vi "RemoteControl.TestLauncher.Client4.vi"() -> ()   [LabVIEW 2016, in "RemoteControl.v2.lvclass"]
uses:
  RemoteControl.v2.lvclass
  <vilib>/JKI/JKI SMO/SMO/Typedefs/SMOState --Enum.ctl
  Typedefs/Message--Cluster.ctl
  C:/Program Files (x86)/National Instruments/LabVIEW 2016/vi.lib/JKI/JKI SMO/SMO/SMO.lvclass
  RemoteControl.STM/RemoteControl.STM.lvclass
  C:/user/patrick/hg/levylab_inst/lvsrc/SMOs/RemoteControl/RemoteControl.v2.lvclass
  Typedefs/PrivateEvents--RemoteControl.SendMessageToProcess.ctl
  <vilib>/JKI/JKI SMO/SMO/SMO.lvclass
panel:
  out "x-y":u32
  out "receive time":u32
  out "send time":u32
  in  "Send":bool
  out "received":i32
  out "sent":i32
  out "Message Sent":T1
  out "Message Received":T1
  in  "T = STM":bool
  in  "Message to Send":T1
  in  "Port":u32=6341
  in  "Address":string
  out "SMO State":T2
  out "error out":errorcluster
  in  "Stop":bool
  # "SM SMO Test Launcher: Client 4"
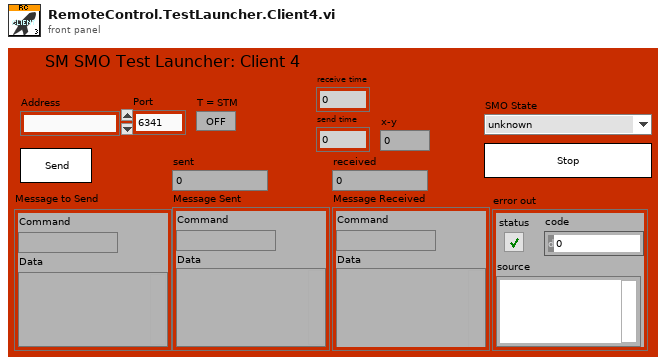
[diagram p1: front panel]
types:
  T1 = typedef "RemoteControl.v2.lvclass/Message--Cluster.ctl" = cluster{"Command":string, "Data":variant}
  T2 = typedef "SMO.lvclass/SMOState --Enum.ctl" = enum16{"unknown", "Created", "Started", "Stopped"}
  T3 = typedef "SMO.lvclass/Public Events.ctl" = cluster{"Error":refnum<user-event>, "State":refnum<user-event>, "Reserve State":refnum<user-event>}
  T4 = typedef "RemoteControl.v2.lvclass/PublicEvents--Cluster.ctl" = cluster{"SendMessageFromProcess":refnum<user-event>}
  T5 = typedef "RemoteControl.v2.lvclass/PrivateEvents--RemoteControl.SendMessageToProcess.ctl" = cluster{"Message":T1, "Message ID":u32}
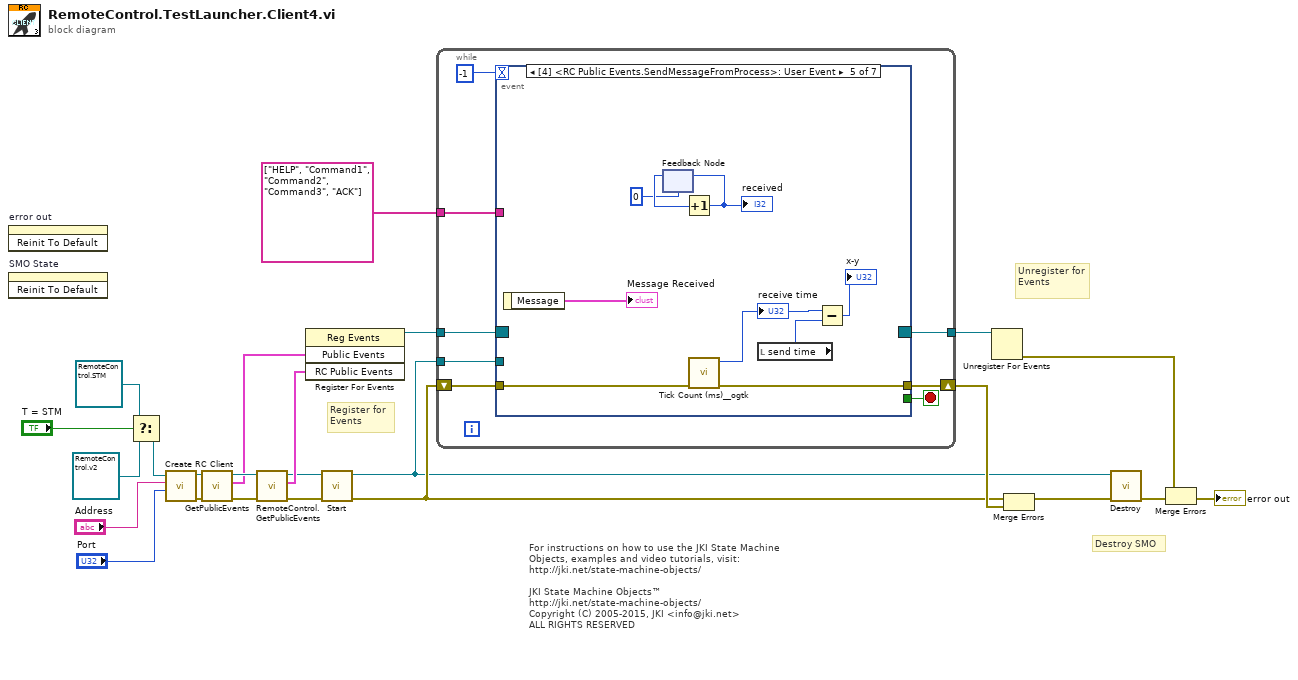
[diagram p0: block diagram]
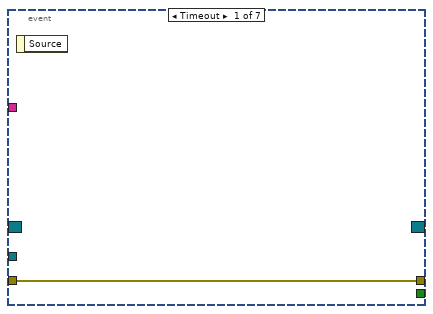
[diagram p2: hidden frame]
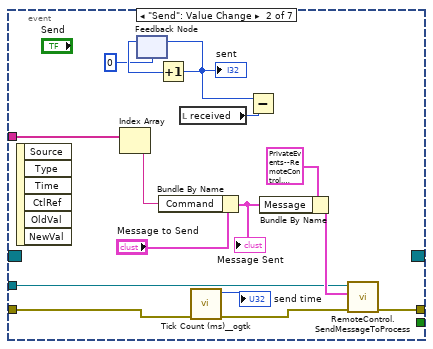
[diagram p3: hidden frame]
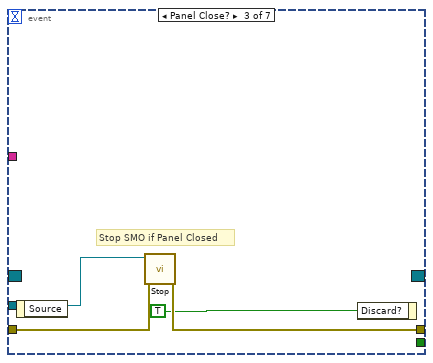
[diagram p4: hidden frame]
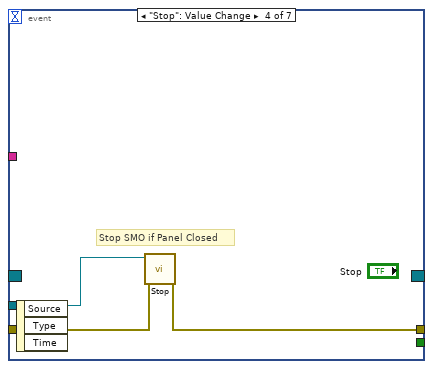
[diagram p5: hidden frame]
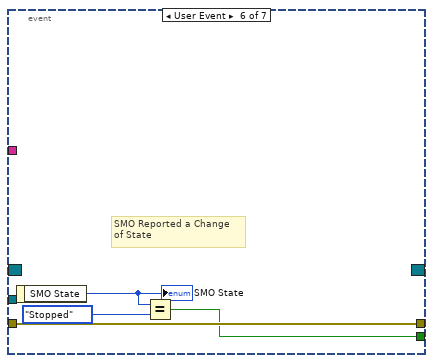
[diagram p6: hidden frame]
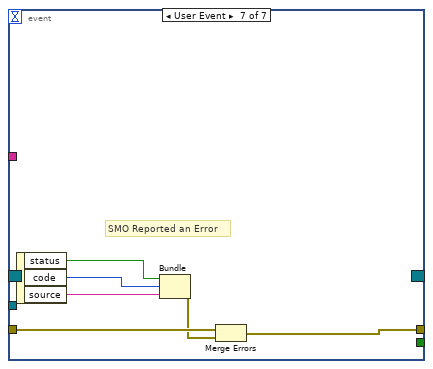
[diagram p7: hidden frame]
diagram:
  # "For instructions on how to use the JKI State Machine Objects, examples and video tutorials, visit:\nhttp://jki.net/state-machine-objects/\n\nJKI State Machine Objects™\nhttp://jki.net/state-machine-objects/\nCopyright (C) 2005-2015, JKI <info@jki.net>\nALL RIGHTS RESERVED"
  # "Destroy SMO"
  # "Unregister for Events"
  # "Register for Events"
  n1 = invoke on="error out" class="Clust (strict)" method="Reinit To Default"() -> ()  [unwired: 3 in, 3 out]
  n2 = invoke on="SMO State" class="Enum (strict)" method="Reinit To Default"() -> ()  [unwired: 3 in, 3 out]
  n3 = Select(t=refnum<class "RemoteControl.STM.lvclass"> refnum ("RemoteControl.STM.lvclass"), s="T = STM", f=refnum<class "RemoteControl.v2.lvclass"> refnum ("SMO.Template.lvclass")) -> (s? t:f=w13:refnum<class "RemoteControl.v2.lvclass">)
  n4 = call-dynamic "Create RC Client.vi"("Port"="Port", "Address"="Address", "RemoteControl in"=w13) -> ("error out"=w12:errorcluster, "RemoteControl out"=w11:refnum<class "RemoteControl.v2.lvclass">)  [unwired: 7 in]
  n5 = call <vilib>:"GetPublicEvents.vi"("error in (no error)"=w12, "SMO"=w11) -> ("error out"=w9:errorcluster, "Public Events"=w8:T3, "SMO out"=w10:refnum<class "RemoteControl.v2.lvclass">)  [unwired: 7 in]
  n6 = call "RemoteControl.GetPublicEvents.vi"("error in (no error)"=w9, "RemoteControl"=w10) -> ("error out"=w4:errorcluster, "RC Public Events"=w7:T4, "RemoteControl out"=w5:refnum<class "RemoteControl.v2.lvclass">)  [unwired: 7 in]
  n7 = register-events(w8, w7) -> (reference out=w6:refnum<event-registration>)  [unwired: 2 in, 1 out]
  n8 = call <vilib>:"Start.vi"("error in (no error)"=w4, "SMO"=w5) -> ("error out"=w3:errorcluster, "SMO out"=w2:refnum<class "RemoteControl.v2.lvclass">)  [unwired: 8 in]
  n9 = while {
    shift-right: [w31] -> w23
    shift-left: w3 -> [w30]
    tunnel: w6 -> [w29]
    tunnel: [w28] -> w24
    tunnel: w2 -> [w27]
    tunnel: string[] ["HELP", "Command1", "Command2", "Command3", "ACK"] ("Commands") -> [w26]
    stop <- w32 stop-if-true
    n10 = event shown="[4] <RC Public Events.SendMessageFromProcess>: User Event" {
      selector: w29 -> [_ _ _ _ _ _ _]
      dyn-events: [_ _ _ _ _ _ _] -> w28
      timeout: -1 -> [_ _ _ _ _ _ _]
      tunnel: [_ _ _ _ _ w65 _] -> w32
      tunnel: w27 -> [_ w38 w52 w55 _ _ _]
      tunnel: [w33 w39 w51 w54 w59 w68 w72] -> w31
      tunnel: w30 -> [w33 w36 w50 w53 w60 w68 w70]
      tunnel: w26 -> [_ w40 _ _ _ _ _]
      event Timeout {
        n11 = event-data() -> ()  [unwired: 1 in, 1 out]
      }
      event "Send": Value Change {
        n12 = event-data() -> ()  [unwired: 1 in, 6 out]
        n13 = Index Array(array=w40) -> (element=w37:string)  [unwired: 1 in]
        n14 = feedback #1(0) -> (w44:i32)
        n15 = Increment(x=w44) -> (x+1=w41:i32)
        "sent" <- w41
        n16 = feedback-in #1(w41) -> ()
        n17 = Bundle By Name(cluster="Message to Send", "Command"=w37) -> (w46:T1)
        "Message Sent" <- w46
        n18 = local read "received"() -> (w42:i32)
        n19 = call <userlib>:"Tick Count (ms)__ogtk.vi"("error in (no error)"=w36) -> ("error out"=w35:errorcluster, "millisecond timer value"=→"send time":u32)  [unwired: 9 in]
        n20 = Subtract(x=w41, y=w42) -> ()  [unwired: 1 out]
        n21 = Bundle By Name(cluster=T5 {"Message"={"Command"="", "Data"=variant(bool FALSE)}, "Message ID"=0} ("SendMessgaeToProcess"), "Message"=w46) -> (w47:T5)
        n22 = call "RemoteControl.SendMessageToProcess.vi"("error in (no error)"=w35, "SendMessgaeToProcess"=w47, "RemoteControl"=w38) -> ("error out"=w39:errorcluster)  [unwired: 7 in, 1 out]
      }
      event Panel Close? {
        # "Stop SMO if Panel Closed"
        n23 = event-data() -> ()  [unwired: 1 in, 1 out]
        n24 = call <vilib>:"Stop.vi"("error in (no error)"=w50, "SMO"=w52) -> ("error out"=w51:errorcluster)  [unwired: 8 in, 1 out]
        n25 = event-data("Discard?"=TRUE ("OK")) -> ()  [unwired: 1 in, 1 out]
      }
      event "Stop": Value Change {
        # "Stop SMO if Panel Closed"
        n26 = event-data() -> ()  [unwired: 1 in, 3 out]
        n27 = call <vilib>:"Stop.vi"("error in (no error)"=w53, "SMO"=w55) -> ("error out"=w54:errorcluster)  [unwired: 8 in, 1 out]
      }
      event User Event {
        n28 = event-data() -> ("Message"=→"Message Received":T1)  [unwired: 1 in]
        n29 = feedback #2(0) -> (w62:i32)
        n30 = Increment(x=w62) -> (x+1=w63:i32)
        "received" <- w63
        n31 = feedback-in #2(w63) -> ()
        n32 = call <userlib>:"Tick Count (ms)__ogtk.vi"("error in (no error)"=w60) -> ("error out"=w59:errorcluster, "millisecond timer value"=w56:u32)  [unwired: 9 in]
        "receive time" <- w56
        n33 = local read "send time"() -> (w58:u32)
        n34 = Subtract(x=w56, y=w58) -> (x-y=→"x-y":u32)
      }
      event User Event {
        # "SMO Reported a Change\nof State"
        n35 = event-data() -> ("SMO State"=w67:T2)  [unwired: 1 in]
        "SMO State" <- w67
        n36 = Equal?(x=w67, y=SMOState_--Enum."Stopped") -> (x = y?=w65:bool)
      }
      event User Event {
        # "SMO Reported an Error"
        n37 = event-data() -> ("status"=w71:bool, "code"=w74:i32, "source"=w73:string)  [unwired: 1 in]
        n38 = Bundle("status"=w71, "code"=w74, "source"=w73) -> (w69:errorcluster)  [unwired: 1 in]
        n39 = Merge Errors(w70, w69) -> (w72:errorcluster)
      }
    }
  }
  n40 = Unregister For Events(event registration refnum=w24) -> (error out=w22:errorcluster)  [unwired: 1 in]
  n41 = Merge Errors(w3, w23) -> (w19:errorcluster)
  n42 = call <vilib>:"Destroy.vi"("error in (no error)"=w19, "SMO"=w2) -> ("error out"=w20:errorcluster)  [unwired: 9 in]
  n43 = Merge Errors(w22, w20) -> (→"error out":errorcluster)
